vi "Get Position Count.vi"(8 "error in (no error)":errorcluster) -> (0 "error out":errorcluster, 3 "Position Count":i32)   [LabVIEW 2011]
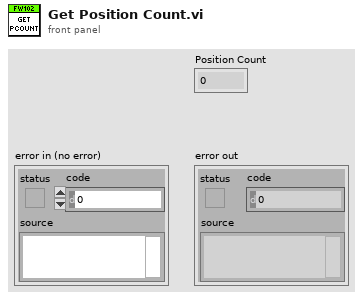
[diagram p1: front panel]
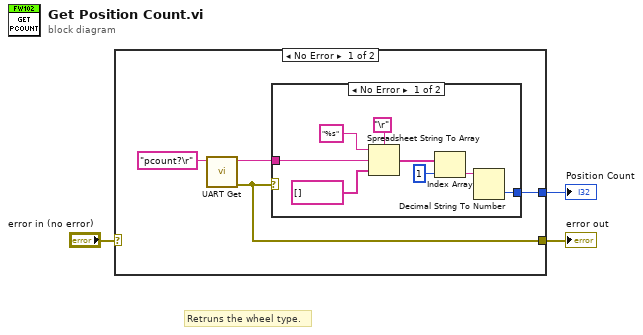
[diagram p0: block diagram]
diagram:
  # "Retruns the wheel type."
  n1 = case shown="No Error" "error in (no error)" {
    selector: "error in (no error)" -> [_ w16]
    tunnel: [w7 w16] -> w3
    tunnel: [w6 _] -> w2
    frame No Error {
      n2 = call "UART Get.vi"("Command"="pcount?\r" ("Input Command String")) -> ("error out"=w7:errorcluster, "Returned String"=w4:string)  [unwired: 9 in]
      n3 = case shown="No Error" w7 {
        tunnel: w4 -> [w15 _]
        tunnel: [w8 _] -> w6
        frame No Error {
          n4 = Spreadsheet String To Array(delimiter (Tab)="\r", format string="%s", spreadsheet string=w15, array type (2D Dbl)=string[] []) -> (array=w11:string[])
          n5 = Index Array(array=w11, index=1) -> (element=w9:string)
          n6 = Decimal String To Number(string=w9) -> (number=w8:i32)  [unwired: 2 in, 1 out]
        }
        frame Error {
        }
      }
    }
    frame Error {
    }
  }
  "error out" <- w3
  "Position Count" <- w2
